vi "Get Sub-Entry DefaultValue+.vi"(8 "Error In":errorcluster, 10 "Sub-Index":u16, 11 "reference in":refnum<class "OD Entry.lvclass">) -> (0 "Error Out":errorcluster, 1 "Found?":bool, 2 "DefaultValue":string, 3 "reference out":refnum<class "OD Entry.lvclass">)   [LabVIEW 2019, in "Electronic Datasheet.lvlib" / "OD Entry.lvclass"]
doc: "Returns default value for a subindex"
uses:
  OD Entry.lvclass
  OD Sub-Entry/OD Sub-Entry.lvclass
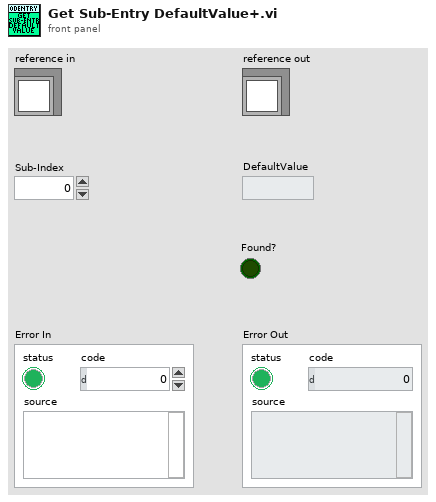
[diagram p1: front panel]
types:
  T1 = typedef "Electronic Datasheet.lvlib/OD Entry.lvclass/ObjectAttributes.ctl" = cluster{"Index":u16, "ObjectType":refnum<class "Object Type Base.lvclass">, "Denotation":string, "Count":u8, "ObjExtend":u8, "Label":string, "Description":string, "PDO Mapping Type":T2, "Sub-Entries":map{u8, refnum<class "OD Sub-Entry.lvclass">}}
  T2 = typedef "Electronic Datasheet.lvlib/PDO Mapping Type.ctl" = enum16{"no", "optional", "RPDO", "TPDO", "UNKNOWN"}
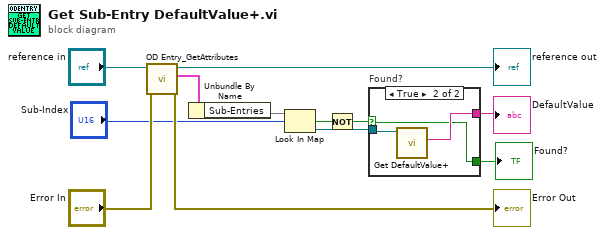
[diagram p0: block diagram]
diagram:
  n1 = call "OD Entry_GetAttributes.vi"("Error In"="Error In", "reference in"="reference in") -> ("Error Out"=→"Error Out":errorcluster, "Data"=w8:T1, "reference out"=→"reference out":refnum<class "OD Entry.lvclass">)  [unwired: 6 in, 1 out]
  n2 = Unbundle By Name(w8) -> ("Sub-Entries"=w7:map{u8, refnum<class "OD Sub-Entry.lvclass">})
  n3 = Look In Map(map=w7, key="Sub-Index") -> (key not found?=w5:bool, value=w4:refnum<class "OD Sub-Entry.lvclass">)  [unwired: 1 in]
  n4 = Not(x=w5) -> (.not. x?=w1:bool)
  n5 = case "Found?" shown="True" w1 {
    selector: w1 -> [w13 w14]
    tunnel: w4 -> [_ w16]
    tunnel: [_ w15] -> w3
    tunnel: [w13 w14] -> w2
    frame False {
    }
    frame True {
      n6 = call "Get DefaultValue+.vi"("reference in"=w16) -> ("DefaultValue"=w15:string)  [unwired: 7 in, 3 out]
    }
  }
  "DefaultValue" <- w3
  "Found?" <- w2
